vi "Output Rate Limiter.vi"(0 "input (controller output)":dbl format="%.2f", 1 "initial output":dbl format="%.2f", 2 "output rate (EGU/min.)":dbl=60.0 format="%.2f", 3 "cycle time (sec.)":dbl=-1.0 format="%.2f", 4 "iteration":i32) -> (5 "output":dbl format="%.2f")   [LabVIEW 2020, in "NI_PID__prctrl compat.lvlib"]
doc: "This function can be used to specify a maximum rate of change of the controller output. Place this VI immediately after the PID VI in your control application.\n\nThe input \"output rate (EGU/min.)\" is used to specify the maximum rate of change of the controller output. The \"iteration\" and \"cycle time (sec.)\" inputs should be the same as those used for the PID VI."
uses:
  NI_PID__prctrl compat.lvlib
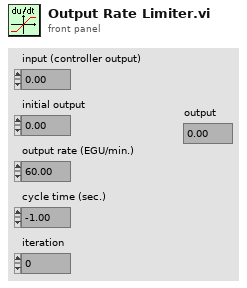
[diagram p1: front panel]
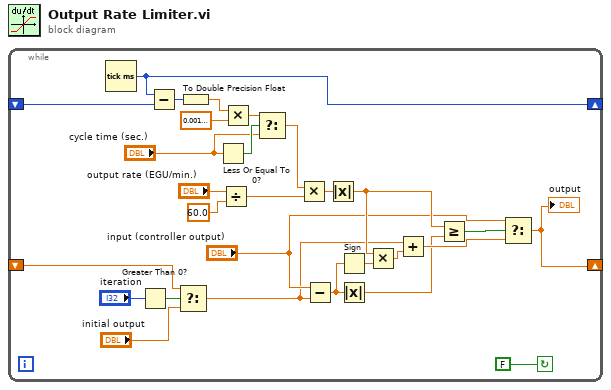
[diagram p0: block diagram]
diagram:
  n1 = while {
    shift-left: _ -> [w17]
    shift-right: [w16] -> _
    shift-left: _ -> [w3]
    shift-right: [w11] -> _
    stop <- FALSE continue-if-true
    n2 = Tick Count (ms)() -> (millisecond timer value=w16:u32)
    n3 = Greater Than 0?(x="iteration") -> (x > 0?=w27:bool)
    n4 = Subtract(x=w16, y=w17) -> (x-y=w20:u32)
    n5 = Select(t=w3, s=w27, f="initial output") -> (s? t:f=w2:dbl)
    n6 = To Double Precision Float(number=w20) -> (double precision float=w21:dbl)
    n7 = Less Or Equal To 0?(x="cycle time (sec.)") -> (x <= 0?=w23:bool)
    n8 = Divide(x="output rate (EGU/min.)", y=60.0) -> (x/y=w14:dbl)
    n9 = Multiply(x=w21, y=0.0010000000474974513) -> (x*y=w22:dbl)
    n10 = Select(t=w22, s=w23, f="cycle time (sec.)") -> (s? t:f=w15:dbl)
    n11 = Multiply(x=w15, y=w14) -> (x*y=w13:dbl)
    n12 = Subtract(x="input (controller output)", y=w2) -> (x-y=w10:dbl)
    n13 = Absolute Value(x=w13) -> (abs(x)=w8:dbl)
    n14 = Sign(1:w10) -> (0:w9:dbl)
    n15 = Absolute Value(x=w10) -> (abs(x)=w5:dbl)
    n16 = Multiply(x=w8, y=w9) -> (x*y=w7:dbl)
    n17 = Add(x=w2, y=w7) -> (x+y=w6:dbl)
    n18 = Greater Or Equal?(x=w8, y=w5) -> (x >= y?=w12:bool)
    n19 = Select(t="input (controller output)", s=w12, f=w6) -> (s? t:f=w11:dbl)
    "output" <- w11
  }
